vi "svc_Is X a Factor of Y.vi"(9 "tolerance":dbl=1e-06, 10 "X":dbl=20.0 format="%#_8g", 11 "Y":dbl=1000.0 format="%#_8g") -> (1 "divisible":bool, 2 "integer ratio":dbl=nan, 3 "residual":dbl=nan format="%#_8g")   [LabVIEW 2017]
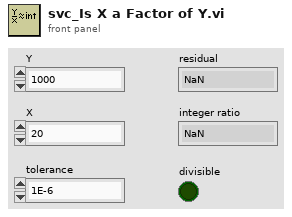
[diagram p1: front panel]
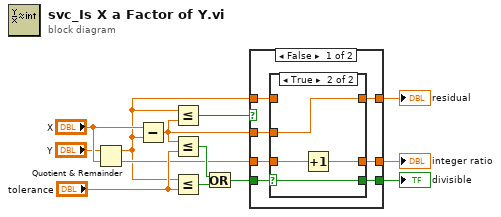
[diagram p0: block diagram]
diagram:
  n1 = Quotient & Remainder(x="Y", y="X") -> (x-y*floor(x/y)=w4:dbl, floor(x/y)=w6:dbl)
  n2 = Subtract(x="X", y=w4) -> (x-y=w2:dbl)
  n3 = Less Or Equal?(x=w4, y=w2) -> (x <= y?=w8:bool)
  n4 = Less Or Equal?(x=w2, y="tolerance") -> (x <= y?=w12:bool)
  n5 = Less Or Equal?(x=w4, y="tolerance") -> (x <= y?=w13:bool)
  n6 = Or(x=w12, y=w13) -> (x .or. y?=w3:bool)
  n7 = case shown="False" w8 {
    tunnel: [w16 w30] -> w7
    tunnel: w6 -> [w18 w30]
    tunnel: [w19 w29] -> w5
    tunnel: w4 -> [w17 w29]
    tunnel: w3 -> [w20 w28]
    tunnel: w2 -> [w15 _]
    tunnel: [w14 w28] -> w1
    frame False {
      n8 = case shown="True" w20 {
        selector: w20 -> [w21 w24]
        tunnel: [w23 w27] -> w19
        tunnel: w18 -> [w22 w26]
        tunnel: w17 -> [w23 _]
        tunnel: [w22 w25] -> w16
        tunnel: w15 -> [_ w27]
        tunnel: [w21 w24] -> w14
        frame False {
        }
        frame True {
          n9 = Increment(x=w26) -> (x+1=w25:dbl)
        }
      }
    }
    frame True {
    }
  }
  "divisible" <- w1
  "residual" <- w5
  "integer ratio" <- w7
